vi "Actor Core.vi"(8 "error in":errorcluster, 11 "UPNCalculator":refnum<class "UPNCalculator.lvclass">) -> (0 "error out":errorcluster, 3 "Actor out":refnum<class "Actor.lvclass">)   [LabVIEW 2012, in "UPNCalculator Actor.lvlib" / "UPNCalculator.lvclass"]
doc: "This is Actor Core.vi, the main message handling loop for Actors. An actor usually just sits in this loop and processes messages as they arrive. Any error returned by the message Do.vi call will stop the loop, with error code 43 as the canonical signal to stop with no error sent to caller. Descendants may override that in Handle Error.vi."
uses:
  UPNCalculator.lvclass
  <vilib>/ActorFramework/Actor/Actor.lvclass
  UPNCalculator Task Msg/UPNCalculator Task Msg.lvclass
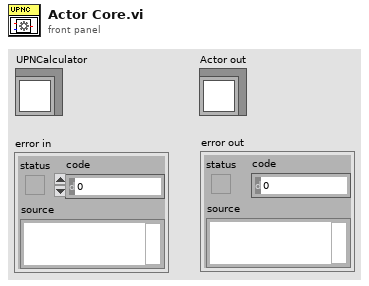
[diagram p1: front panel]
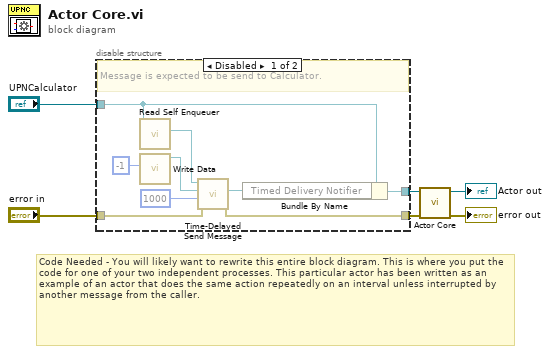
[diagram p0: block diagram]
diagram:
  # "Code Needed - You will likely want to rewrite this entire block diagram. This is where you put the code for one of your two independent processes. This particular actor has been written as an example of an actor that does the same action repeatedly on an interval unless interrupted by another message from the caller."
  n1 = disable-structure shown="Disabled" {
    disable-tunnel: "UPNCalculator" -> [w13 w16]
    disable-tunnel: [w12 w16] -> w3
    disable-tunnel: "error in" -> [w10 w17]
    disable-tunnel: [w9 w17] -> w1
    frame Disabled {
      # "Message is expected to be send to Calculator."
      n2 = call <vilib>:"Read Self Enqueuer.vi"("Actor"=w13) -> ("Self Enqueuer"=w15:refnum<class "Message Enqueuer.lvclass">)  [unwired: 10 in]
      n3 = call "Write Data.vi"("Data"=-1) -> ("UPNCalculator Task Msg out"=w8:refnum<class "UPNCalculator Task Msg.lvclass">)  [unwired: 10 in]
      n4 = call <vilib>:"Time-Delayed Send Message.vi"("error in (no error)"=w10, "Milliseconds To Wait"=1000, "Message"=w8, "Message Enqueuer"=w15) -> ("error out"=w9:errorcluster, "Delivery Notifier"=w11:refnum<notifier>)  [unwired: 6 in]
      n5 = Bundle By Name(cluster=w13, "Timed Delivery Notifier"=w11) -> (w12:refnum<class "UPNCalculator.lvclass">)
    }
    frame Enabled {
      # "To be used with UPNCalculatorGUI"
    }
  }
  n6 = call-parent "Actor Core.vi"("error in"=w1, "Actor in"=w3) -> ("error out"=→"error out":errorcluster, "Actor out"=→"Actor out":refnum<class "Actor.lvclass">)  [unwired: 8 in]
